vi "Intake_teleop.vi"(11 "Joystick_Out":T1) -> ()   [LabVIEW 2020]
uses:
  Intake_control_states.ctl
  Intake_cluster.ctl
  Globals/Intake_Motor_global.vi
  Utility VIs/Joystick_Controls.ctl
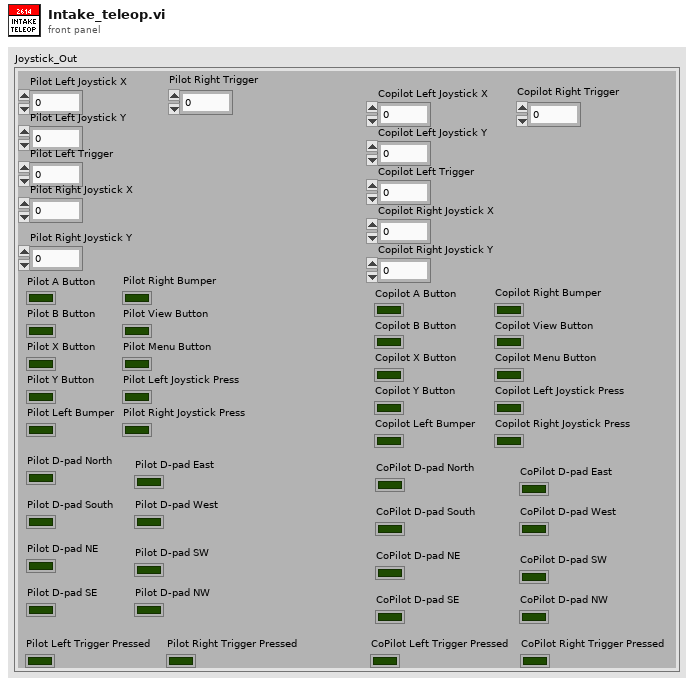
[diagram p1: front panel]
types:
  T1 = typedef "Joystick_Controls.ctl" = cluster{"Pilot Left Joystick X":dbl, "Pilot Left Joystick Y":dbl, "Pilot A Button":bool, "Pilot B Button":bool, "Pilot X Button":bool, "Pilot Y Button":bool, "Pilot Left Bumper":bool, "Pilot Right Bumper":bool, "Pilot View Button":bool, "Pilot Menu Button":bool, "Pilot Left Joystick Press":bool, "Pilot Right Joystick Press":bool, "Pilot Left Trigger":dbl, "Pilot Right Joystick X":dbl, "Pilot Right Joystick Y":dbl, "Pilot Right Trigger":dbl, "Copilot Left Joystick X":dbl, "Copilot Left Joystick Y":dbl, "Copilot A Button":bool, "Copilot B Button":bool, "Copilot X Button":bool, "Copilot Y Button":bool, "Copilot Left Bumper":bool, "Copilot Right Bumper":bool, "Copilot View Button":bool, "Copilot Menu Button":bool, "Copilot Left Joystick Press":bool, "Copilot Right Joystick Press":bool, "Copilot Left Trigger":dbl, "Copilot Right Joystick X":dbl, "Copilot Right Joystick Y":dbl, "Copilot Right Trigger":dbl, "Pilot D-pad North":bool, "Pilot D-pad South":bool, "Pilot D-pad East":bool, "Pilot D-pad West":bool, "Pilot D-pad NE ":bool, "Pilot D-pad SE":bool, "Pilot D-pad SW":bool, "Pilot D-pad NW":bool, "CoPilot D-pad North":bool, "CoPilot D-pad South":bool, "CoPilot D-pad East":bool, "CoPilot D-pad West":bool, "CoPilot D-pad NE":bool, "CoPilot D-pad SE":bool, "CoPilot D-pad SW":bool, "CoPilot D-pad NW":bool, "Pilot Left Trigger Pressed":bool, "Pilot Right Trigger Pressed":bool, "CoPilot Left Trigger Pressed":bool, "CoPilot Right Trigger Pressed":bool}
  T2 = typedef "Intake_cluster.ctl" = cluster{"control_states":T3, "Manual_control":dbl, "Trigger?":bool}
  T3 = typedef "Intake_control_states.ctl" = enum16{"Manual_op", "No_Op"}
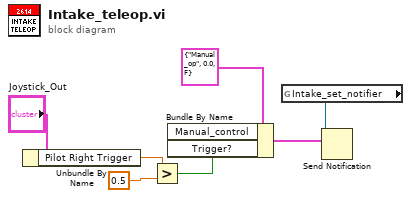
[diagram p0: block diagram]
diagram:
  n1 = Unbundle By Name("Joystick_Out") -> ("Pilot Right Trigger"=w4:dbl)
  n2 = Greater?(x=w4, y=0.5) -> (0:w5:bool)
  n3 = Bundle By Name(cluster=T2 {"control_states"=enum."Manual_op", "Manual_control"=0.0, "Trigger?"=FALSE} ("Intake_cluster"), "Trigger?"=w5) -> (w6:T2)  [unwired: 1 in]
  n4 = global read "Intake_Motor_global.vi" "Intake_set_notifier"() -> (w7:refnum<notifier>)
  n5 = Send Notification(notification=w6, notifier=w7) -> ()  [unwired: 1 in, 2 out]
